vi "CloseSF.vi"(0 "connection IDs":T1) -> ()   [LabVIEW 2010]
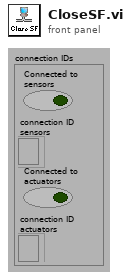
[diagram p1: front panel]
types:
  T1 = cluster{"Connected to\nsensors":bool, "connection ID\nsensors":refnum<k5>, "Connected to\nactuators":bool, "connection ID\nactuators":refnum<k5>}
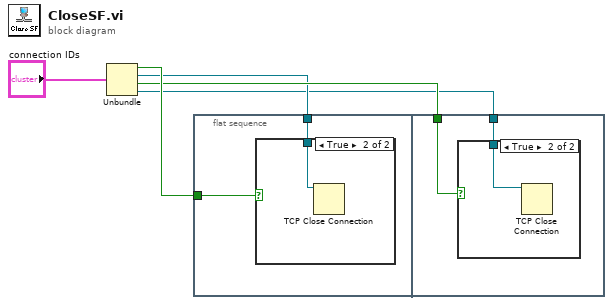
[diagram p0: block diagram]
diagram:
  n1 = Unbundle("connection IDs") -> ("Connected to\nsensors"=w4:bool, "connection ID\nsensors"=w2:refnum<k5>, "Connected to\nactuators"=w3:bool, "connection ID\nactuators"=w1:refnum<k5>)
  n2 = flat-sequence {
    tunnel: w4 -> [w7]
    tunnel: w2 -> [w6]
    tunnel: w3 -> [w10]
    tunnel: w1 -> [w9]
    frame #0 {
      n3 = case shown="True" w7 {
        tunnel: w6 -> [_ w8]
        frame False {
        }
        frame True {
          n4 = TCP Close Connection(connection ID=w8) -> ()  [unwired: 2 in, 2 out]
        }
      }
    }
    frame #1 {
      n5 = case shown="True" w10 {
        tunnel: w9 -> [_ w11]
        frame False {
        }
        frame True {
          n6 = TCP Close Connection(connection ID=w11) -> ()  [unwired: 2 in, 2 out]
        }
      }
    }
  }
